vi "start_sweep.vi"(8 "error in (no error)":errorcluster, 11 "StimulatorDL090727DAQmx in":refnum<class "StimulatorDL090727Writer.lvclass">) -> (0 "error out":errorcluster, 3 "StimulatorDL090727DAQmx out":refnum<class "StimulatorDL090727Writer.lvclass">)   [LabVIEW 2010, in "StimulatorDL090727Writer.lvclass"]
uses:
  StimulatorDL090727Writer.lvclass
  StimulatorDL090727Writer.lvclass/StimulatorDL090727Writer.ctl
  SignalWriter/GenericSignalWriter/GenericSignalWriter/GenericSignalWriter.lvclass
  StimulatorDL090724Scaffold/StimulatorDL090724Scaffold/Stimulator090724Scaffold.lvclass
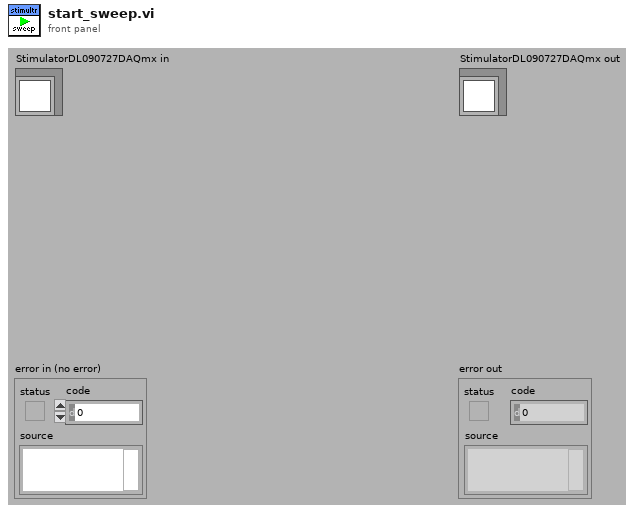
[diagram p1: front panel]
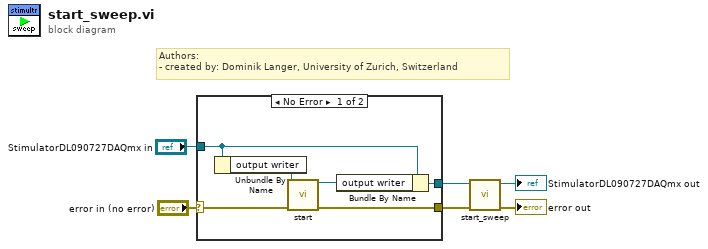
[diagram p0: block diagram]
diagram:
  # "Authors: \n- created by: Dominik Langer, University of Zurich, Switzerland"
  n1 = case shown="No Error" "error in (no error)" {
    selector: "error in (no error)" -> [w10 w14]
    tunnel: [w9 w14] -> w1
    tunnel: [w11 w13] -> w3
    tunnel: "StimulatorDL090727DAQmx in" -> [w12 w13]
    frame No Error {
      n2 = Unbundle By Name(w12) -> ("output writer"=w8:refnum<class "GenericSignalWriter.lvclass">)
      n3 = call-dynamic "start.vi"("error in (no error)"=w10, "WriteSignalsGenericPlugin in"=w8) -> ("error out"=w9:errorcluster, "WriteSignalsGenericPlugin out"=w7:refnum<class "GenericSignalWriter.lvclass">)  [unwired: 8 out]
      n4 = Bundle By Name(cluster=w12, "output writer"=w7) -> (w11:refnum<class "StimulatorDL090727Writer.lvclass">)
    }
    frame Error {
    }
  }
  n5 = call-parent "start_sweep.vi"("error in (no error)"=w1, "Stimulator090724Scaffold in"=w3) -> ("error out"=→"error out":errorcluster, "Stimulator090724Scaffold out"=→"StimulatorDL090727DAQmx out":refnum<class "StimulatorDL090727Writer.lvclass">)  [unwired: 8 in]
